vi "CRYCal eq & corr curves paths.vi"(0 "Calibrated Device Name":string, 5 "Channel Name":string, 7 "In_Out":bool) -> (3 "Sens Currve Name":string, 4 "Sens Curve File":string, 6 "Corr Curve Name":string, 8 "Corr Curve File":string, 10 "EQ Curve Name":string, 15 "EQ Curve File":string)   [LabVIEW 2013]
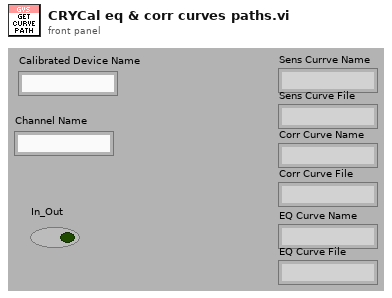
[diagram p1: front panel]
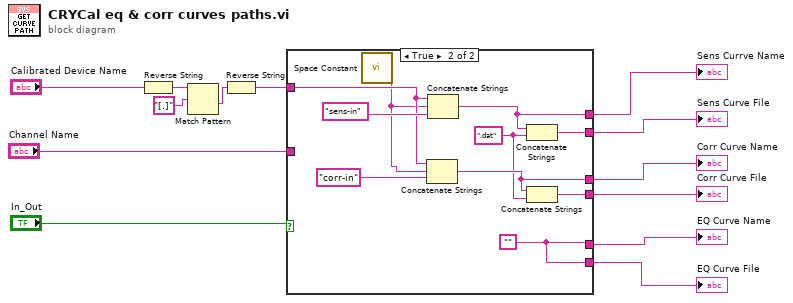
[diagram p0: block diagram]
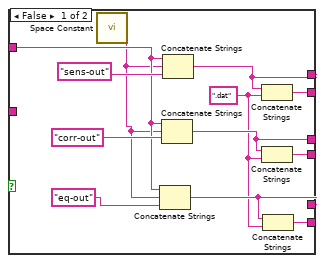
[diagram p2: hidden frame]
diagram:
  n1 = Reverse String(1:"Calibrated Device Name") -> (0:w5:string)
  n2 = Match Pattern(string=w5, regular expression="[.]") -> (after substring=w3:string)  [unwired: 4 out]
  n3 = Reverse String(1:w3) -> (0:w1:string)
  n4 = case shown="True" "In_Out" {
    tunnel: w1 -> [w19 w34]
    tunnel: "Channel Name" -> [_ _]
    tunnel: [w23 w31] -> w11
    tunnel: [w21 w29] -> w9
    tunnel: [w22 w30] -> w10
    tunnel: [w20 w27] -> w8
    tunnel: [w16 w26] -> w7
    tunnel: [w14 w26] -> w6
    frame False {
      w15 = ".dat"
      n5 = call <vilib>:"Space Constant.vi"() -> ("String"=w18:string)
      n6 = Concatenate Strings(w19, w18, "eq-out") -> (w16:string)
      n7 = Concatenate Strings(w19, w18, "corr-out") -> (w21:string)
      n8 = Concatenate Strings(w19, w18, "sens-out") -> (w23:string)
      n9 = Concatenate Strings(w23, w15) -> (w22:string)
      n10 = Concatenate Strings(w21, w15) -> (w20:string)
      n11 = Concatenate Strings(w16, w15) -> (w14:string)
    }
    frame True {
      w26 = ""
      w28 = ".dat"
      n12 = call <vilib>:"Space Constant.vi"() -> ("String"=w32:string)
      n13 = Concatenate Strings(w34, w32, "corr-in") -> (w29:string)
      n14 = Concatenate Strings(w34, w32, "sens-in") -> (w31:string)
      n15 = Concatenate Strings(w31, w28) -> (w30:string)
      n16 = Concatenate Strings(w29, w28) -> (w27:string)
    }
  }
  "Sens Currve Name" <- w11
  "Sens Curve File" <- w10
  "Corr Curve Name" <- w9
  "Corr Curve File" <- w8
  "EQ Curve Name" <- w7
  "EQ Curve File" <- w6
